vi "CallDeviceSubViDynamic.vi"(4 "device conneced":bool, 6 "error in":errorcluster, 8 "State Queue":string, 9 "Data cluster":T1) -> (0 "error out":errorcluster, 1 "states out":string, 3 "Data cluster out":T1)   [LabVIEW 2009]
uses:
  dataCluster.ctl
  <vilib>/vision/Image Controls.llb/IMAQ Image.ctl
  DataQueueTypeDef.ctl
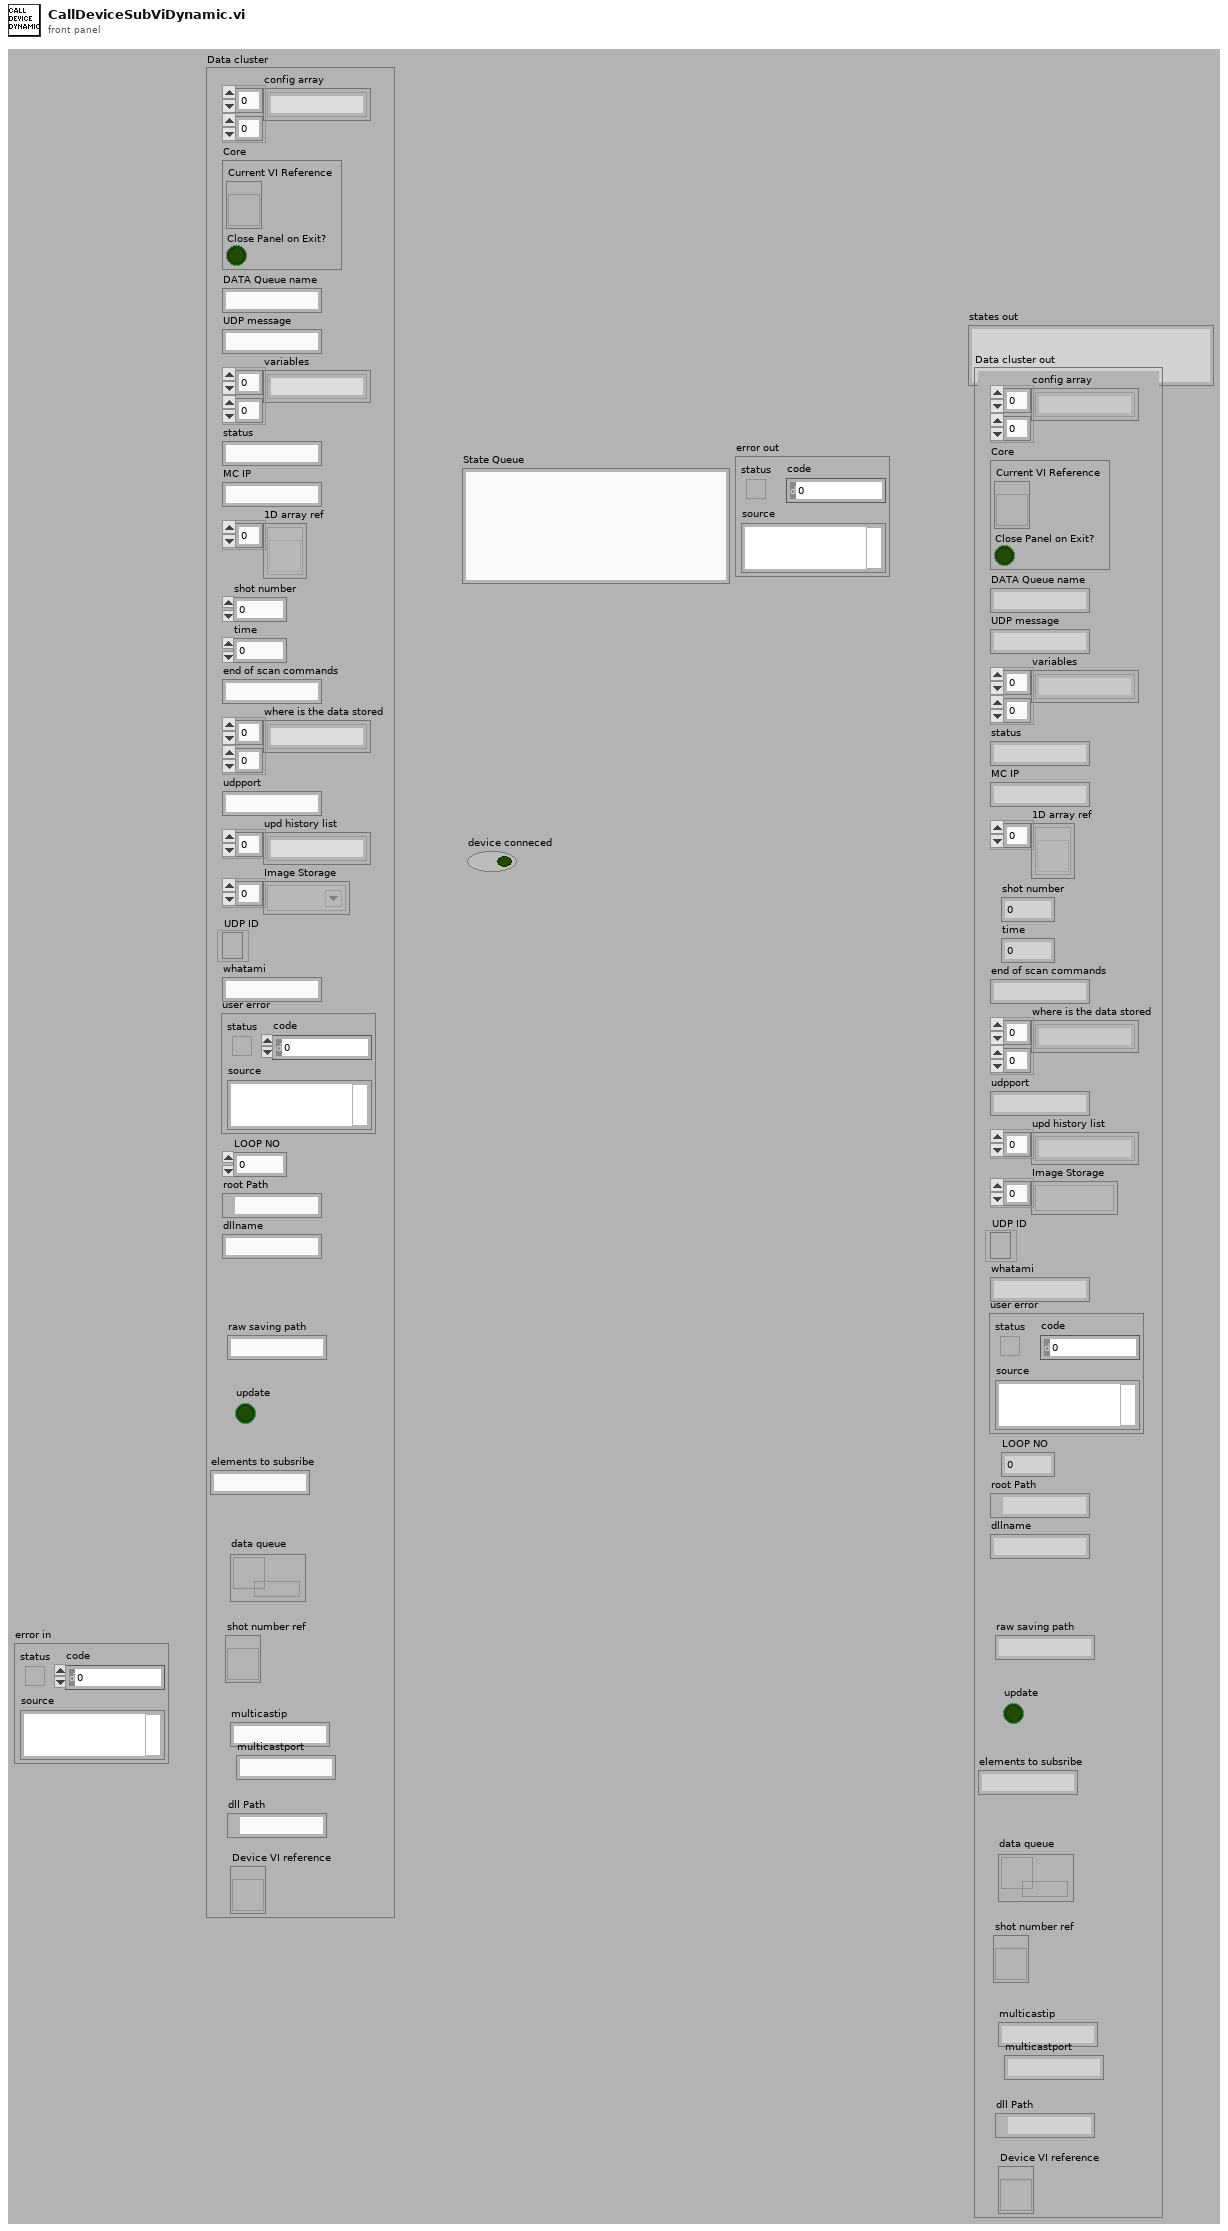
[diagram p1: front panel]
types:
  T1 = typedef "dataCluster.ctl" = cluster{"config array":string[][], "Core":cluster{"Current VI Reference":refnum<vi>, "Close Panel on Exit?":bool}, "DATA Queue name":string, "UDP message":string, "variables":string[][], "status":string, "MC IP":string, "1D array ref":refnum<vi>[], "shot number":i32, "time":u32, "end of scan commands":string, "where is the data stored":string[][], "udpport":string, "upd history list":string[], "Image Storage":T2[], "UDP ID":refnum<k16>, "whatami":string, "user error":errorcluster, "LOOP NO":u32, "root Path":path, "dllname":string, "raw saving path":string, "update":bool, "elements to subsribe":string, "data queue":refnum<queue>, "shot number ref":refnum<vi>, "multicastip":string, "multicastport":string, "dll Path":path, "Device VI reference":refnum<vi>}
  T2 = typedef "IMAQ Image.ctl" = refnum<image>
  T3 = cluster{"config array":string[][], "where is the data stored":string[][], "variables":string[][], "1D array ref":refnum<vi>[], "Image Storage":string[], "Settings":string[][]}
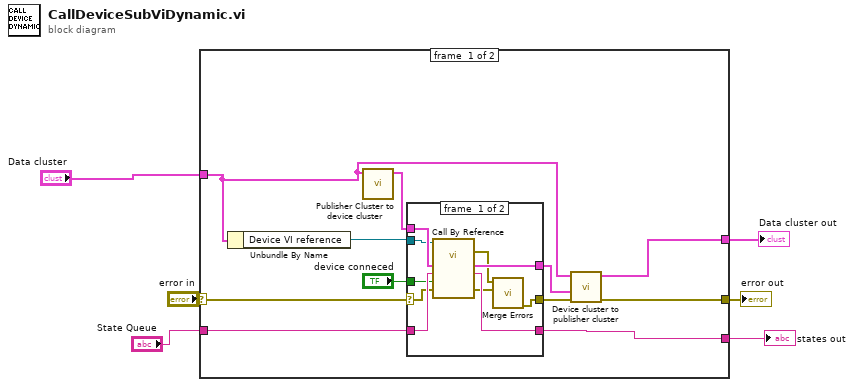
[diagram p0: block diagram]
diagram:
  n1 = case shown="No Error" "error in" {
    selector: "error in" -> [w12 w33]
    tunnel: [w13 w33] -> w6
    tunnel: [w11 w31] -> w4
    tunnel: "State Queue" -> [w10 w31]
    tunnel: [w9 w32] -> w2
    tunnel: "Data cluster" -> [w8 w32]
    frame #0 {
      n2 = Unbundle By Name(w8) -> ("Device VI reference"=w7:refnum<vi>)
      n3 = call "Publisher Cluster to device cluster.vi"("publisher cluster"=w8) -> ("Device cluster"=w17:T3)  [unwired: 10 in]
      n4 = case shown="No Error" w12 {
        selector: w12 -> [w18 w28]
        tunnel: w17 -> [w27 w30]
        tunnel: w10 -> [w26 w29]
        tunnel: "device conneced" -> [w25 _]
        tunnel: [w24 w30] -> w15
        tunnel: [w23 w29] -> w11
        tunnel: [w19 w28] -> w14
        tunnel: w7 -> [w22 _]
        frame #0 {
          n5 = call-by-ref "?"(reference=w22, "error in"=w18, "device conneced"=w25, "State Queue"=w26, "Device cluster"=w27) -> (error out=w21:errorcluster, 0:"error out"=w20:errorcluster, "States Out"=w23:string, "Device cluster out"=w24:T3)  [unwired: 6 in, 1 out]
          n6 = call <vilib>:"Merge Errors.vi"("error in 2 (no error)"=w20, "error in 1 (no error)"=w21) -> ("error out"=w19:errorcluster)  [unwired: 5 in]
        }
        frame #1 {
        }
      }
      n7 = call "Device cluster to publisher cluster.vi"("error in"=w14, "Device cluster from subVi/Dll"=w15, "old Data cluster"=w8) -> ("errorout"=w13:errorcluster, "Data cluster out"=w9:T1)  [unwired: 7 in]
    }
    frame #1 {
    }
  }
  "error out" <- w6
  "states out" <- w4
  "Data cluster out" <- w2
